vi "ShiftRegisterExample.vi"() -> ()   [LabVIEW 2018]
panel:
  out "Value Appended to Array":dbl
  in  "stop":bool
  out "Element":dbl
  in  "index":i32
  out "Current Loop Iteration":dbl
  out "Array Indicator 2":dbl[](array[numeric])
  out "Array Indicator 1":dbl[](array[numeric])
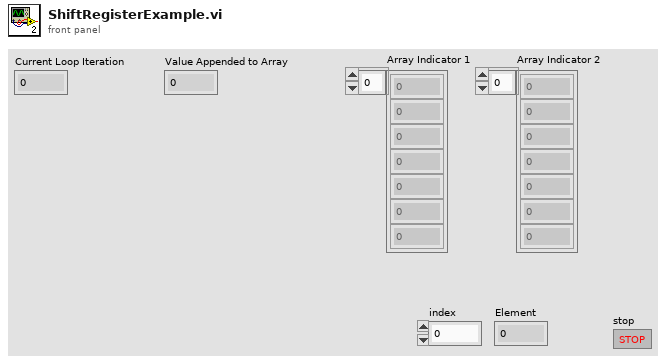
[diagram p1: front panel]
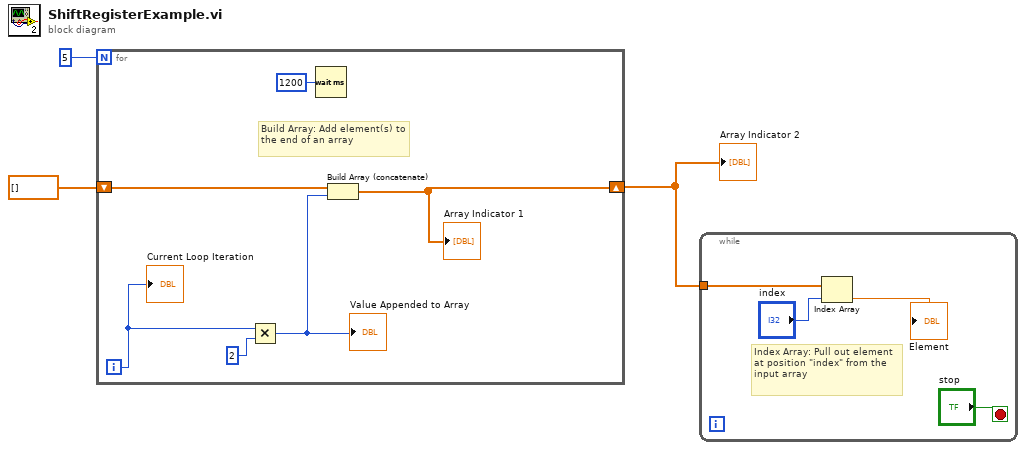
[diagram p0: block diagram]
diagram:
  n1 = for {
    N: 5 ("Numeric") -> [_]
    shift-right: [w7] -> w1
    shift-left: dbl[] [] ("Array 3") -> [w8]
    i -> [w5]
    # "Build Array: Add element(s) to the end of an array"
    n2 = Multiply(x=w5, y=2) -> (x*y=w4:i32)
    "Value Appended to Array" <- w4
    n3 = Wait (ms)(milliseconds to wait=u32 1200) -> ()  [unwired: 1 out]
    n4 = Build Array (concatenate)(w8, w4) -> (w7:dbl[])
    "Array Indicator 1" <- w7
    "Current Loop Iteration" <- w5
  }
  "Array Indicator 2" <- w1
  n5 = while {
    tunnel: w1 -> [w13]
    stop <- "stop" stop-if-true
    # "Index Array: Pull out element at position \"index\" from the input array"
    n6 = Index Array(array=w13, index="index") -> (element=→"Element":dbl)
  }
